vi "Get Params.vi"(8 "error in (no error)":errorcluster, 10 "Log Class":refnum<class "Build_Javier_Lopez_lib_Configuration_Filejson class.lvclass">, 11 "Module Launcher Base in":refnum<class "Launcher Base.lvclass">) -> (0 "error out":errorcluster, 3 "Module Launcher Base out":refnum<class "Launcher Base.lvclass">)   [LabVIEW 2021, in "Launcher Base.lvclass"]
uses:
  Launcher Base.lvclass
  <vilib>/Javier Lopez/Configuration File/Json Element/Build_Javier_Lopez_lib_Configuration_Filejson class.lvclass
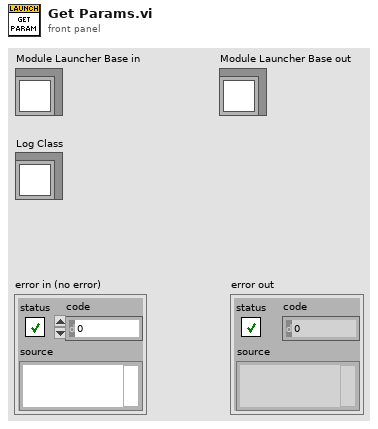
[diagram p1: front panel]
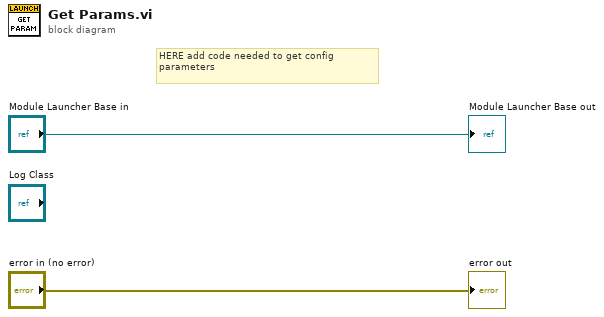
[diagram p0: block diagram]
diagram:
  # "HERE add code needed to get config\nparameters"
  "error out" <- "error in (no error)"
  "Module Launcher Base out" <- "Module Launcher Base in"
